vi "Test Matrix Type.vi"   [LabVIEW 2024, in "NI_AALPro.lvlib"]
doc: "<p>Tests whether<strong> Input Matrix</strong> is a matrix of special type. Wire data to the <strong>Input Matrix</strong> input to determine the polymorphic instance to use or <a href=\"nihelplauncher://docs/csh?context=lvcore_lvhowto_selectingdefaultinstpolyvi\">manually select</a> the instance.</p>"
uses:
  NI_AALPro.lvlib
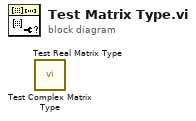
[diagram p0: block diagram]
diagram:
  n1 = call "Test Complex Matrix Type.vi"() -> ()  [unwired: 10 in, 2 out]
  n2 = call "Test Real Matrix Type.vi"() -> ()  [unwired: 10 in, 2 out]
